vi "PQconninfoFree.vi"(8 "error in (no error)":errorcluster, 11 "connOptions":T1) -> (0 "error out":errorcluster, 3 "connOptions out":T1)   [LabVIEW 2019, in "libpqlv.lvlib"]
uses:
  libpqlv.lvlib
  libpq.dll
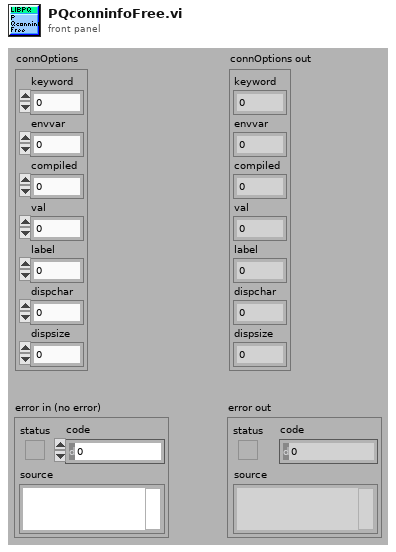
[diagram p1: front panel]
types:
  T1 = cluster{"keyword":u32, "envvar":u32, "compiled":u32, "val":u32, "label":u32, "dispchar":u32, "dispsize":i32}
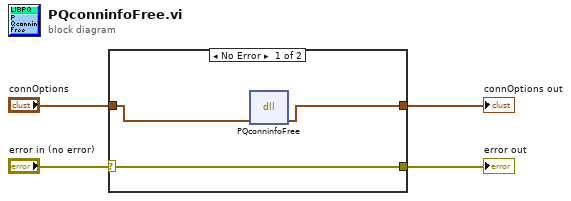
[diagram p0: block diagram]
diagram:
  n1 = case shown="No Error" "error in (no error)" {
    selector: "error in (no error)" -> [w7 w9]
    tunnel: [w7 w9] -> w3
    tunnel: "connOptions" -> [w6 w8]
    tunnel: [w5 w8] -> w1
    frame No Error {
      n2 = dll-call lib="libpq.*" fn="PQconninfoFree"("connOptions"=w6) -> ("connOptions"=w5:T1)  [unwired: 4 in, 2 out]
    }
    frame Error {
    }
  }
  "connOptions out" <- w1
  "error out" <- w3
